vi "ffmpegger.vi"() -> ()   [LabVIEW 2020]
panel:
  in  "Tab Control":enum32{"Input", "Progress", "Diagnostics"}(tab)
  out "fileSizes":i64[](array[numeric]) format="%_3p"
  in  "paths":path[](array[path])
  in  "Output directory (Dialogue if blank)":path
  in  "Input type":enum32{"Item 0", "Item 1"}(radio)
  in  "Slowdown":dbl=4.0
  in  "LinearSizeReduction":dbl=2.0
  out "Progress (by completed bytes)":dbl(slide) scale=0.0..1.0
  out "Start Time":timestamp format="%<%b-%d %H:%M>T"
  out "Progress":string
  out "Predicted Completion":timestamp format="%<%b-%d %H:%M>T"
  out "CompletionPrediction":dbl(graph)
  out "Results":T1(array[cluster])
  out "bytes/sec":dbl format="%_3p"
  out "totalBytes":i64 format="%#_4p"
  in  "fileTypes":string="*.mp4;*.mov;*.m4v"
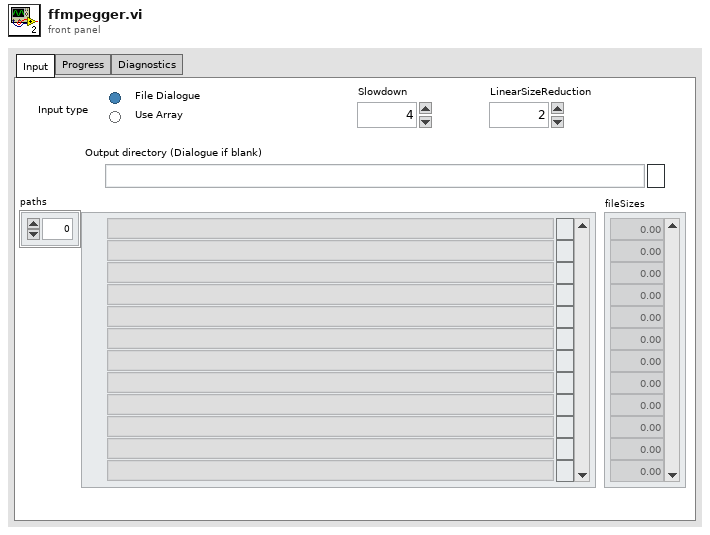
[diagram p1: front panel]
types:
  T1 = cluster{"standard error":string, "standard output":string, "return code":i32, "error out":errorcluster}[]
  T2 = cluster{"standard output":string, "standard error":string, "return code":i32, "error out":errorcluster}[]
  T3 = cluster{"standard output":string, "standard error":string, "return code":i32, "error out":errorcluster}
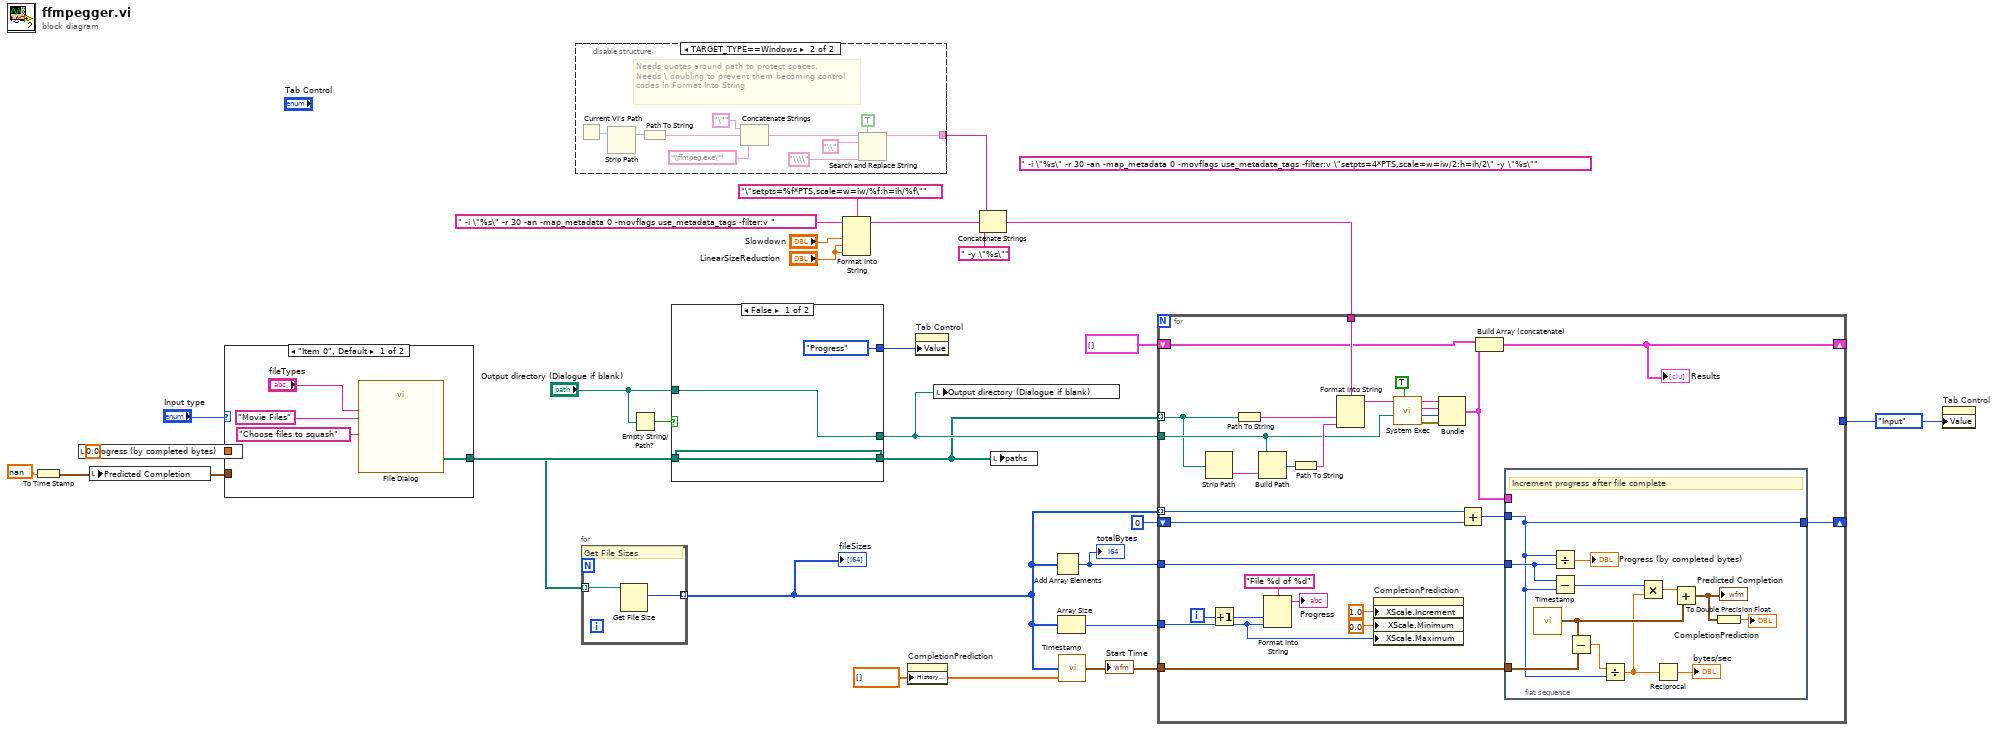
[diagram p0: block diagram]
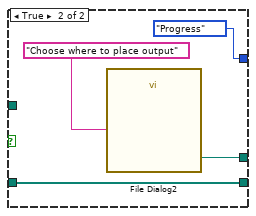
[diagram p2: hidden frame]
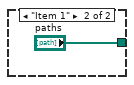
[diagram p3: hidden frame]
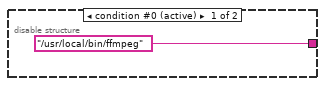
[diagram p4: hidden frame]
diagram:
  w2 = dbl[] [] ("History Data")
  w3 = enum32{"Input", "Progress", "Diagnostics"}."Input" ("Tab Control")
  w8 = 0.0 ("Progress (by size)")
  (unwired) " -i \"%s\" -r 30 -an -map_metadata 0 -movflags use_metadata_tags -filter:v \"setpts=4*PTS,scale=w=iw/2:h=ih/2\" -y \"%s\"" ("format string")
  n1 = To Time Stamp(1:nan) -> (0:w7:timestamp)
  n2 = local write "Progress (by completed bytes)"(w8) -> ()
  n3 = local write "Predicted Completion"(w7) -> ()
  n4 = case shown="\"Item 0\", Default" "Input type" {
    tunnel: [w30 "paths"] -> w11
    tunnel: w8 -> [_ _]
    tunnel: w7 -> [_ _]
    frame "Item 0", Default {
      n5 = call "File Dialog"("prompt"="Choose files to squash", "pattern (all files)"="fileTypes", "pattern label"="Movie Files") -> ("selected paths"=w30:path[])  [unwired: 9 in, 3 out]
    }
    frame "Item 1" {
    }
  }
  n6 = disable-structure shown="TARGET_TYPE==Windows" {
    disable-tunnel: ["/usr/local/bin/ffmpeg" ("format string") w37] -> w20
    frame condition #0 (active) {
    }
    frame condition #1 {
      # "Needs quotes around path to protect spaces. Needs \\ doubling to prevent them becoming control codes in Format Into String"
      n7 = Current VI's Path() -> (path=w41:path)
      n8 = Strip Path(path=w41) -> (stripped path=w40:path)  [unwired: 1 out]
      n9 = Path To String(path=w40) -> (string=w39:string)
      n10 = Concatenate Strings("\"" ("format string"), w39, "\\ffmpeg.exe\"" ("format string")) -> (w36:string)
      n11 = Search and Replace String(replace all?=TRUE ("replace all? (F)"), input string=w36, search string="\\", replace string="\\\\" ("replace string (\"\")")) -> (result string=w37:string)  [unwired: 4 in, 3 out]
    }
  }
  n12 = Empty String/Path?(string/path="Output directory (Dialogue if blank)") -> (empty?=w24:bool)
  n13 = case shown="False" w24 {
    tunnel: [w45 w49] -> w21
    tunnel: "Output directory (Dialogue if blank)" -> [w45 _]
    tunnel: [w44 w47] -> w6
    tunnel: w11 -> [w44 w47]
    tunnel: [enum32{"Input", "Progress", "Diagnostics"}."Progress" ("Tab Control") enum32{"Input", "Progress", "Diagnostics"}."Progress" ("Tab Control")] -> w4
    frame False {
    }
    frame True {
      n14 = call "File Dialog2"("prompt"="Choose where to place output") -> ("selected path"=w49:path)  [unwired: 11 in, 3 out]
    }
  }
  n15 = for {
    tunnel: w6 -> [w51] mode=indexing
    tunnel: [w50] -> w1 mode=indexing
    # "Get File Sizes"
    n16 = Get File Size(file=w51) -> (size (in bytes)=w50:i64)  [unwired: 1 in, 2 out]
  }
  "fileSizes" <- w1
  n17 = Format Into String(format string="\"setpts=%f*PTS,scale=w=iw/%f:h=ih/%f\"", initial string=" -i \"%s\" -r 30 -an -map_metadata 0 -movflags use_metadata_tags -filter:v " ("format string"), "Slowdown", "LinearSizeReduction", "LinearSizeReduction") -> (resulting string=w17:string)  [unwired: 1 in, 1 out]
  n18 = property on="CompletionPrediction" class="WFChart (strict)"("History Data"=w2) -> ()  [unwired: 2 in, 2 out]
  n19 = property on="Tab Control" class="TabCtl (strict)"("Value"=w4) -> ()  [unwired: 2 in, 2 out]
  n20 = local write "Output directory (Dialogue if blank)"(w21) -> ()
  n21 = Concatenate Strings(w20, w17, " -y \"%s\"" ("format string")) -> (w26:string)
  n22 = local write "paths"(w6) -> ()
  n23 = Add Array Elements(numeric array=w1) -> (sum=w19:i64)
  "totalBytes" <- w19
  n24 = Array Size(array=w1) -> (size(s)=w5:i32)
  n25 = call "Timestamp.vi"("Anything 3"=w2, "Anything 2"=w1) -> ("Start Time"=w10:timestamp)  [unwired: 3 in]
  "Start Time" <- w10
  n26 = for {
    tunnel: w6 -> [w69] mode=indexing
    tunnel: w21 -> [w74]
    tunnel: w26 -> [w76]
    shift-right: [w64] -> _
    shift-left: T2 [] -> [w68]
    shift-right: [w63] -> _
    shift-left: i64 0 -> [w58]
    tunnel: w1 -> [w57] mode=indexing
    tunnel: w19 -> [w66]
    tunnel: w10 -> [w65]
    tunnel: w5 -> [w54]
    tunnel: w3 -> [_]
    i -> [w62]
    n27 = Strip Path(path=w69) -> (name=w79:string)  [unwired: 1 out]
    n28 = Increment(x=w62) -> (x+1=w55:i32)
    n29 = Path To String(path=w69) -> (string=w80:string)
    n30 = Build Path(base path=w74, name or relative path=w79) -> (appended path=w78:path)
    n31 = Format Into String(format string="File %d of %d", w55, w54) -> (resulting string=→"Progress":string)  [unwired: 2 in, 1 out]
    n32 = Path To String(path=w78) -> (string=w77:string)
    n33 = Format Into String(format string=w76, w80, w77) -> (resulting string=w75:string)  [unwired: 2 in, 1 out]
    n34 = property on="CompletionPrediction" class="WFChart (strict)"("XScale.Increment"=1.0 ("X Scale.Range:Increment"), "XScale.Minimum"=0.0 ("X Scale.Range:Minimum"), "XScale.Maximum"=w54) -> ()  [unwired: 2 in, 2 out]
    n35 = call <vilib>:"System Exec.vi"("wait until completion? (T)"=TRUE, "working directory"=w74, "command line"=w75) -> ("error out"=w70:errorcluster, "return code"=w71:i32, "standard error"=w72:string, "standard output"=w73:string)  [unwired: 5 in]
    n36 = Bundle("standard output"=w73, "standard error"=w72, "return code"=w71, "error out"=w70) -> (w59:T3)  [unwired: 1 in]
    n37 = Add(x=w57, y=w58) -> (x+y=w56:i64)
    n38 = Build Array (concatenate)(w68, w59) -> (w64:T2)
    "Results" <- w64
    n39 = flat-sequence {
      tunnel: w66 -> [w91]
      tunnel: w65 -> [w90]
      tunnel: [w81] -> w63
      tunnel: w59 -> [_]
      tunnel: w56 -> [w81]
      frame #0 {
        # "Increment progress after file complete"
        n40 = call "Timestamp.vi"() -> ("Start Time"=w86:timestamp)  [unwired: 5 in]
        n41 = Divide(x=w81, y=w91) -> (x/y=→"Progress (by completed bytes)":dbl)
        n42 = Subtract(x=w91, y=w81) -> (x-y=w88:i64)
        n43 = Subtract(x=w86, y=w90) -> (x-y=w89:dbl)
        n44 = Divide(x=w89, y=w81) -> (x/y=w85:dbl)
        n45 = Multiply(x=w88, y=w85) -> (x*y=w87:dbl)
        n46 = Reciprocal(x=w85) -> (1/x=→"bytes/sec":dbl)
        n47 = Add(x=w87, y=w86) -> (x+y=w83:timestamp)
        "Predicted Completion" <- w83
        n48 = To Double Precision Float(number=w83) -> (double precision float=→"CompletionPrediction":dbl)
      }
    }
  }
  n49 = property on="Tab Control" class="TabCtl (strict)"("Value"=w3) -> ()  [unwired: 2 in, 2 out]
